vi "Read.vi"(8 "error in (no error)":errorcluster, 11 "One Terminal in":refnum<class "AbsFunc_One Term_STR.lvclass">) -> (0 "error out":errorcluster, 2 "String":string, 3 "One Terminal out":refnum<class "AbsFunc_One Term_STR.lvclass">)   [LabVIEW 2021, in "AbsFunc_One Term_STR.lvclass"]
uses:
  AbsFunc_One Term_STR.lvclass
  AbsFunc_One Term_STR.lvclass/AbsFunc_One Term_STR.ctl
  Abs_Types/String/Abs_String.lvclass
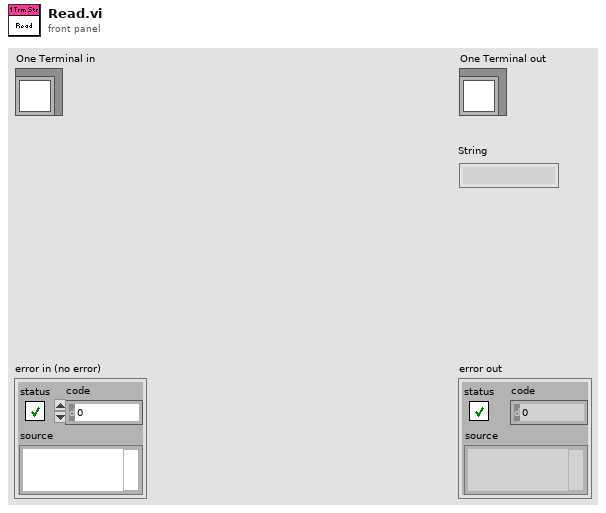
[diagram p1: front panel]
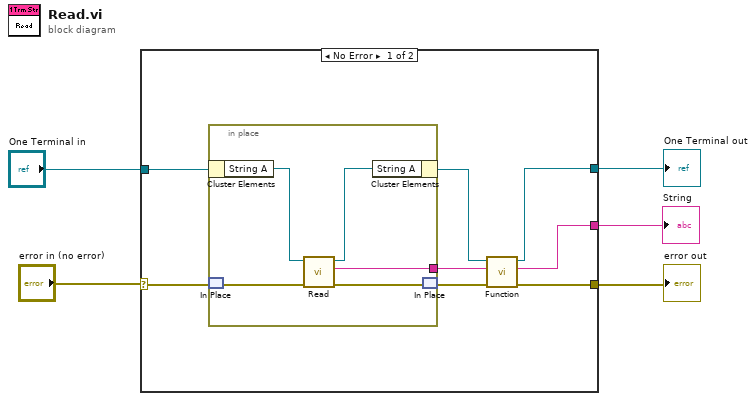
[diagram p0: block diagram]
diagram:
  n1 = case shown="No Error" "error in (no error)" {
    selector: "error in (no error)" -> [w13 w19]
    tunnel: "One Terminal in" -> [w12 w20]
    tunnel: [w8 w20] -> w3
    tunnel: [w7 w19] -> w2
    tunnel: [w6 _] -> w1
    frame No Error {
      n2 = in-place {
        in-place-border: [w14] -> w9
        n3 = in-place-cluster #1(w12) -> ("String A"=w16:refnum<class "Abs_String.lvclass">)
        n4 = in-place-match #2(w13) -> (w18:errorcluster)
        n5 = call-dynamic "Read.vi"("error in (no error)"=w18, "Abs_String in"=w16) -> ("error out"=w17:errorcluster, "String"=w14:string, "Abs_String out"=w15:refnum<class "Abs_String.lvclass">)  [unwired: 7 in]
        n6 = in-place-cluster #1("String A"=w15) -> (w10:refnum<class "AbsFunc_One Term_STR.lvclass">)
        n7 = in-place-match #2(w17) -> (w11:errorcluster)
      }
      n8 = call-dynamic "Function.vi"("error in (no error)"=w11, "String A"=w9, "One Terminal in"=w10) -> ("error out"=w7:errorcluster, "String"=w6:string, "One Terminal out"=w8:refnum<class "AbsFunc_One Term_STR.lvclass">)  [unwired: 6 in]
    }
    frame Error {
    }
  }
  "error out" <- w2
  "One Terminal out" <- w3
  "String" <- w1
